vi "get channels from mapping set.vi"(10 "channel classification":T4, 11 "mappings set":T1[](array[typedef])) -> (3 "channels":refnum<class "TBM channel.lvclass">[](array[class]))   [LabVIEW 2013, in "engine configuration.lvclass"]
uses:
  engine configuration.lvclass
  <vilib>/NI/Tag Bus Module Framework/channel/TBM channel.lvclass
  <vilib>/NI/Tag Bus Module Framework/channel/channel classification.ctl
  <vilib>/NI/Tag Bus/table/mapping specification.ctl
  <vilib>/NI/Tag Bus/tag/Data Type.ctl
  <vilib>/NI/Tag Bus/table/mapping.ctl
  <vilib>/NI/Tag Bus/tag/tag descriptor.lvclass/tag descriptor.ctl
  <vilib>/NI/Tag Bus Module Framework/channel/TBM channel.lvclass/TBM channel.ctl
  <vilib>/NI/Tag Bus/tag/write tag name.vi
  <vilib>/NI/Tag Bus/tag/write data type.vi
  <vilib>/NI/Tag Bus Module Framework/channel/Write channel classification.vi
  <vilib>/NI/Tag Bus/tag/tag descriptor.lvclass
  <vilib>/NI/Tag Bus/table/data table.lvlib
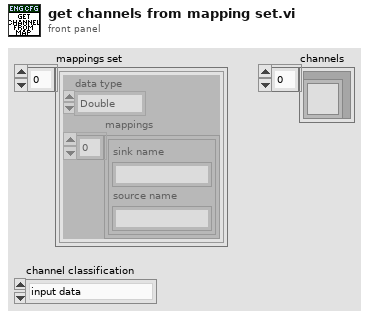
[diagram p1: front panel]
types:
  T1 = typedef "tag bus.lvlib/data table.lvlib/mapping specification.ctl" = cluster{"data type":T2, "mappings":T3[]}
  T2 = typedef "tag bus.lvlib/tag descriptor.lvclass/Data Type.ctl" = enum16{"Double", "Single", "I64", "I32", "I16", "I8", "U64", "U32", "U16", "U8", "Boolean", "String", "Array of Double", "Array of Single", "Array of I64", "Array of I32", "Array of I16", "Array of I8", "Array of U64", "Array of U32", "Array of U16", "Array of U8", "Array of Boolean", "Array of String"}
  T3 = typedef "tag bus.lvlib/data table.lvlib/mapping.ctl" = cluster{"sink name":string, "source name":string}
  T4 = typedef "TBM channel.lvclass/channel classification.ctl" = enum16{"input data", "output data", "processing parameter", "processing result"}
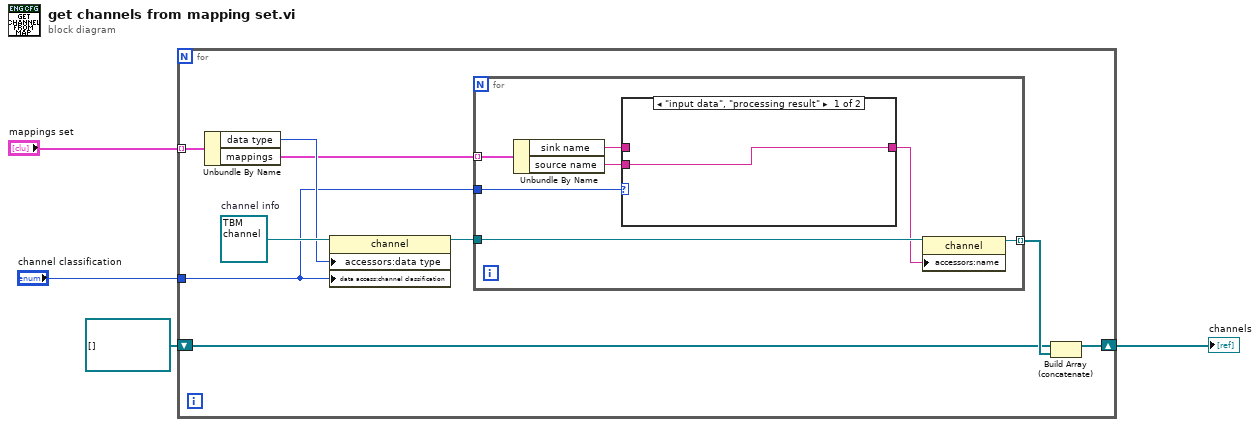
[diagram p0: block diagram]
diagram:
  n1 = for {
    tunnel: "mappings set" -> [w13] mode=indexing
    tunnel: "channel classification" -> [w8]
    shift-right: [w6] -> w4
    shift-left: refnum<class "TBM channel.lvclass">[] [] -> [w5]
    w12 = refnum<class "TBM channel.lvclass"> refnum  # channel info
    n2 = Unbundle By Name(w13) -> ("data type"=w11:T2, "mappings"=w10:T3[])
    n3 = property class="channel"(reference=w12, "accessors:data type"=w11, "data access:channel classification"=w8) -> (reference out=w9:refnum<class "TBM channel.lvclass">)  [unwired: 1 in, 1 out]
    n4 = for {
      tunnel: w10 -> [w20] mode=indexing
      tunnel: w9 -> [w16]
      tunnel: w8 -> [w19]
      tunnel: [w14] -> w7 mode=indexing
      n5 = Unbundle By Name(w20) -> ("sink name"=w18:string, "source name"=w17:string)
      n6 = case shown="\"input data\", \"processing result\"" w19 {
        tunnel: w18 -> [_ w22]
        tunnel: w17 -> [w21 _]
        tunnel: [w21 w22] -> w15
        frame "input data", "processing result" {
        }
        frame "output data", "processing parameter" {
        }
      }
      n7 = property class="channel"(reference=w16, "accessors:name"=w15) -> (reference out=w14:refnum<class "TBM channel.lvclass">)  [unwired: 1 in, 1 out]
    }
    n8 = Build Array (concatenate)(w5, w7) -> (w6:refnum<class "TBM channel.lvclass">[])
  }
  "channels" <- w4
